vi "Turn.vi"   [LabVIEW 2016, in "Moving Motor.lvrbt"]
uses:
  Moving Motor.lvrbt
  <vilib>/NXT/Hardware/Plugins/Tetrix DC Motor/TetrixDCMotorAddress.ctl
  <vilib>/NXT/NXTIO Xnodes/NXTIONodeSubVIs/TETRIX IO Move DC Motors.vi
  <vilib>/NXT/NXTIO Xnodes/NXTIONodeSubVIs/TETRIX IO Stop DC Motors.vi
  <vilib>/NXT/Subs/LVHSConnector.ctl
  <vilib>/NXT/NXTIO Xnodes/AddressXNode/NXTIOAddress.xnode
  <vilib>/NXT/NXTIO Xnodes/NXTIOXNode/NXTIO.xnode
  <vilib>/NXT/LegoClasses/BrickReference/BrickReference.lvclass
types:
  T1 = typedef "TetrixDCMotorAddress.ctl" = i32
  T2 = typedef "LVHSConnector.ctl" = refnum<class "BrickReference.lvclass">
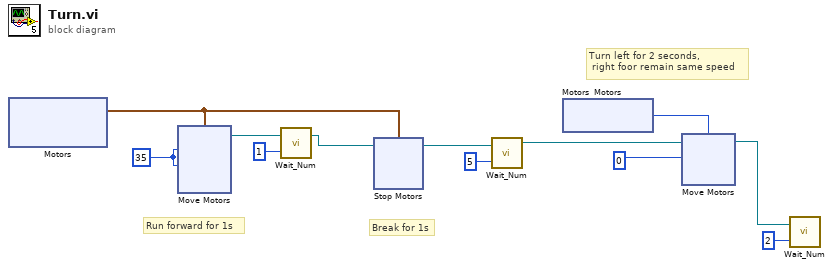
[diagram p0: block diagram]
diagram:
  w12 = 35
  # "Break for 1s"
  # "Run forward for 1s"
  # "Turn left for 2 seconds,\n right foor remain same speed"
  n1 = xnode "Motors"() -> ("Motor"=w6:cluster{"TetrixDCMotor":T1, "TetrixDCMotor":T1})
  n2 = xnode "Move Motors"("Power/Speed 2"=w12, "Power/Speed 1"=w12, "Motors"=w6) -> ("NXT/EV3"=w5:T2)  [unwired: 1 in]
  n3 = call <vilib>:"Wait_Num.vi"("Time (1 sec)"=1, "NXT/EV3"=w5) -> ("NXT/EV3"=w1:T2)  [unwired: 2 in]
  n4 = xnode "Stop Motors"("Motors"=w6, "NXT/EV3"=w1) -> ("NXT/EV3"=w3:T2)
  n5 = call <vilib>:"Wait_Num.vi"("Time (1 sec)"=5, "NXT/EV3"=w3) -> ("NXT/EV3"=w2:T2)  [unwired: 2 in]
  n6 = xnode "Motors"() -> ()  [unwired: 1 out]
  n7 = xnode "Motors"() -> ("Motor"=w10:T1)
  n8 = xnode "Move Motors"("Power/Speed 1"=0, "Motors"=w10, "NXT/EV3"=w2) -> ("NXT/EV3"=w7:T2)
  n9 = call <vilib>:"Wait_Num.vi"("Time (1 sec)"=2, "NXT/EV3"=w7) -> ()  [unwired: 2 in, 1 out]
